vi "Initialize.vi"(8 "error in":errorcluster, 10 "shared resources":refnum<class "Shared Resources.lvclass">, 11 "Rx UDP Execution Unit in":refnum<class "Rx UDP Execution Unit.lvclass">) -> (0 "error out":errorcluster, 3 "Rx UDP Execution Unit out":refnum<class "Rx UDP Execution Unit.lvclass">)   [LabVIEW 2020, in "AIM ARINC 664 Engine.lvlib" / "Implementation.lvlib" / "Rx UDP Execution Unit.lvclass"]
uses:
  Rx UDP Execution Unit.lvclass
  Interfaces/Shared Resources/Shared Resources.lvclass
  Rx UDP Execution Unit.lvclass/Rx UDP Execution Unit.ctl
  <instrlib>/AIM GmbH/_AIM 664/bsp/Fdx Create Session (Rx-VL-Oriented).vi
  <instrlib>/AIM GmbH/_AIM 664/bsp/Receive/FdxCreateRxVL.vi
  <instrlib>/AIM GmbH/_AIM 664/bsp/Fdx Create UDP Port (RX-CommPort).vi
  <instrlib>/AIM GmbH/_AIM 664/AIM664LV.lvlib
  <vilib>/Utility/SystemLogging/NI_SystemLogging.lvlib
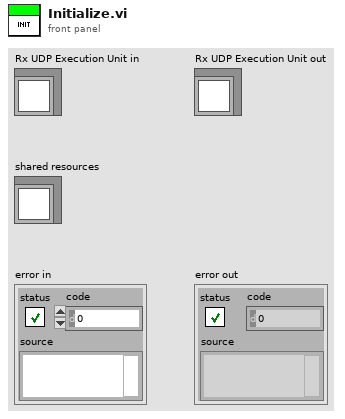
[diagram p1: front panel]
types:
  T1 = typedef "AIM664LV.lvlib/comm_verification_rx.ctl" = cluster{"VlId":u16, "VLRange":u32, "VerificationMode":u32, "Bag":u32, "Jitter":u32, "MaxFrameLength":u32, "MaxSkew":u32, "VLBufSize":u32, "FilterMode":u32, "FilterPosition":u32, "Padding":u32, "FilterMask":u32, "FilterData":u32, "MinFrameLength":u32}
  T2 = typedef "AIM664LV.lvlib/comm_udp_rx.ctl" = cluster{"PortType":enum16{"FDX_UDP_SAMPLING", "FDX_UDP_QUEUING"}, "SubVIId":u32, "domainID":u8, "sideID":u8, "locationID":u8, "partitionID":u8, "UdpSrcPort":u16, "UdpDstPort":u16, "UdpNumBufMessages":u32, "UdpMaxMessageSize":u32, "UdpSamplingRate":u32}
  T3 = cluster{"VL Config":T1, "CommPort Config":T2[]}[]
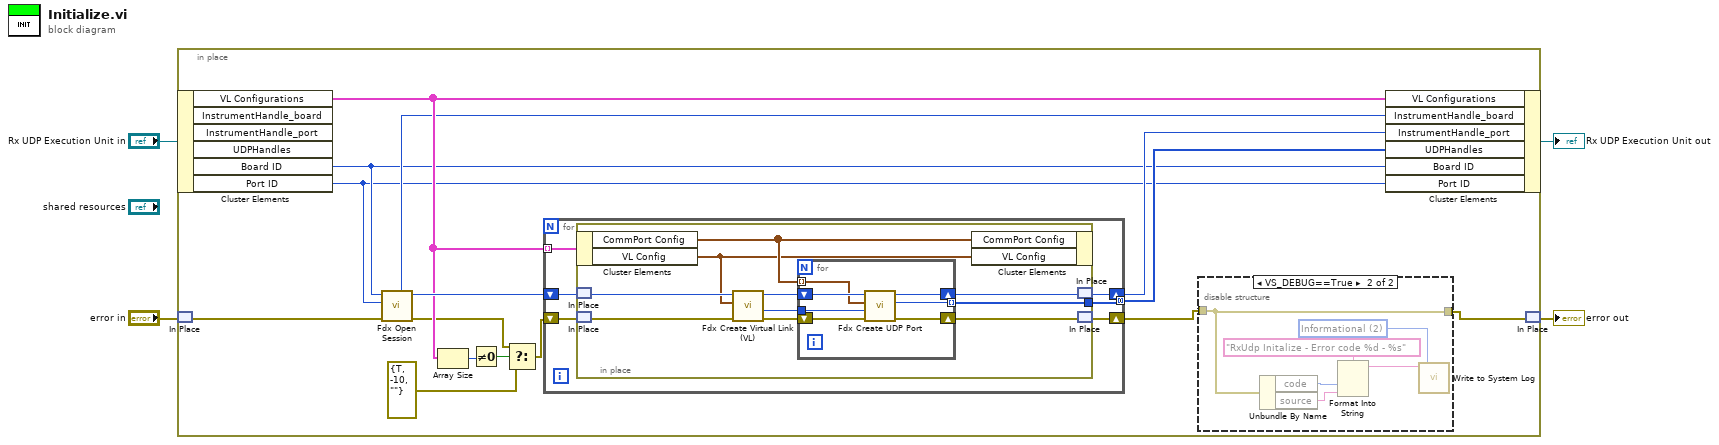
[diagram p0: block diagram]
diagram:
  n1 = in-place {
    n2 = in-place-cluster #1("Rx UDP Execution Unit in") -> ("VL Configurations"=w13:T3, "Board ID"=w8:u32, "Port ID"=w7:u32)  [unwired: 3 out]
    n3 = in-place-match #2("error in") -> (w19:errorcluster)
    n4 = call-poly <instrlib>:"Fdx Open Session.vi"("error in (no error)"=w19, "port"=w7, "board"=w8) -> ("error out"=w10:errorcluster, "InstrumentHandle_port out"=w18:u32, "InstrumentHandle_board out"=w12:u32)  [unwired: 3 in, 3 out]
    n5 = Array Size(array=w13) -> (size(s)=w16:i32)
    n6 = Not Equal To 0?(x=w16) -> (x != 0?=w15:bool)
    n7 = Select(t=w10, s=w15, f=errorcluster {"status"=TRUE, "code"=-10, "source"=""}) -> (s? t:f=w9:errorcluster)
    n8 = for {
      tunnel: w13 -> [w31] mode=indexing
      shift-right: [w29] -> w11
      shift-left: w18 -> [w30]
      shift-right: [w28] -> w6
      shift-left: w9 -> [w32]
      tunnel: [w27] -> w17 mode=concatenating
      n9 = in-place {
        in-place-border: [w34] -> w27
        n10 = in-place-cluster #3(w31) -> ("CommPort Config"=w38:T2[], "VL Config"=w37:T1)
        n11 = in-place-match #4(w30) -> (w41:u32)
        n12 = in-place-match #5(w32) -> (w42:errorcluster)
        n13 = call-poly <instrlib>:"Fdx Create Virtual Link (VL).vi"("error in (no error)"=w42, "VL Config"=w37, "InstrumentHandle_port in"=w41) -> ("error out"=w40:errorcluster, "VlId"=w33:u16, "InstrumentHandle_port out"=w39:u32)  [unwired: 6 in]
        n14 = for {
          shift-right: [w48] -> w36
          shift-left: w40 -> [w49]
          shift-right: [w46] -> w35
          shift-left: w39 -> [w47]
          tunnel: w38 -> [w45] mode=indexing
          tunnel: [w44] -> w34 mode=indexing
          tunnel: w33 -> [w43]
          n15 = call-poly <instrlib>:"Fdx Create UDP Port.vi"("error in"=w49, "VlId"=w43, "CommPort Config"=w45, "port handle in"=w47) -> ("error out"=w48:errorcluster, "commPort handle out"=w44:u32, "port handle out"=w46:u32)  [unwired: 4 in, 1 out]
        }
        n16 = in-place-cluster #3("CommPort Config"=w38, "VL Config"=w37) -> ()  [unwired: 1 out]
        n17 = in-place-match #4(w35) -> (w29:u32)
        n18 = in-place-match #5(w36) -> (w28:errorcluster)
      }
    }
    n19 = disable-structure shown="VS_DEBUG==True" {
      disable-tunnel: w6 -> [w20 w21]
      disable-tunnel: [w20 w21] -> w5
      frame condition #0 (active) {
      }
      frame condition #1 {
        w24 = 2 items=["Error", "Warning", "Informational"] ("severity")
        n20 = Unbundle By Name(w21) -> ("code"=w23:i32, "source"=w22:string)
        n21 = Format Into String(format string="RxUdp Initalize - Error code %d - %s", w23, w22) -> (resulting string=w25:string)  [unwired: 2 in, 1 out]
        n22 = call <vilib>:"Write to System Log.vi"("severity"=w24, "message"=w25) -> ()  [unwired: 9 in, 1 out]
      }
    }
    n23 = in-place-cluster #1("VL Configurations"=w13, "InstrumentHandle_board"=w12, "InstrumentHandle_port"=w11, "UDPHandles"=w17, "Board ID"=w8, "Port ID"=w7) -> (→"Rx UDP Execution Unit out":refnum<class "Rx UDP Execution Unit.lvclass">)
    n24 = in-place-match #2(w5) -> (→"error out":errorcluster)
  }
